vi "AssertDisable.vi"() -> (15 "error out":errorcluster)   [LabVIEW 2016, in "DronaTest.lvlib"]
uses:
  DronaTest.lvlib
  APIs/Stimulus/ControlValue/ValueSignalByPathString.vi
  APIs/Assert/AssertControlDisable/AssertDisabled.vi
  APIs/Assert/AssertControlDisable/AssertDisabledAndGrayedOut.vi
  APIs/Assert/AssertControlDisable/AssertEnabled.vi
  <vilib>/addons/_JKI Toolkits/Caraya/classes/Test/Test.lvclass
  Drona.lvlib
  APIs/Stimulus/ControlValue/ControlValue.lvlib
  APIs/Assert/AssertControlDisable/AssertControlDisable.lvlib
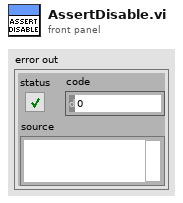
[diagram p1: front panel]
types:
  T1 = enum8{"Enabled", "Disabled", "Disabled and Grayed Out"}
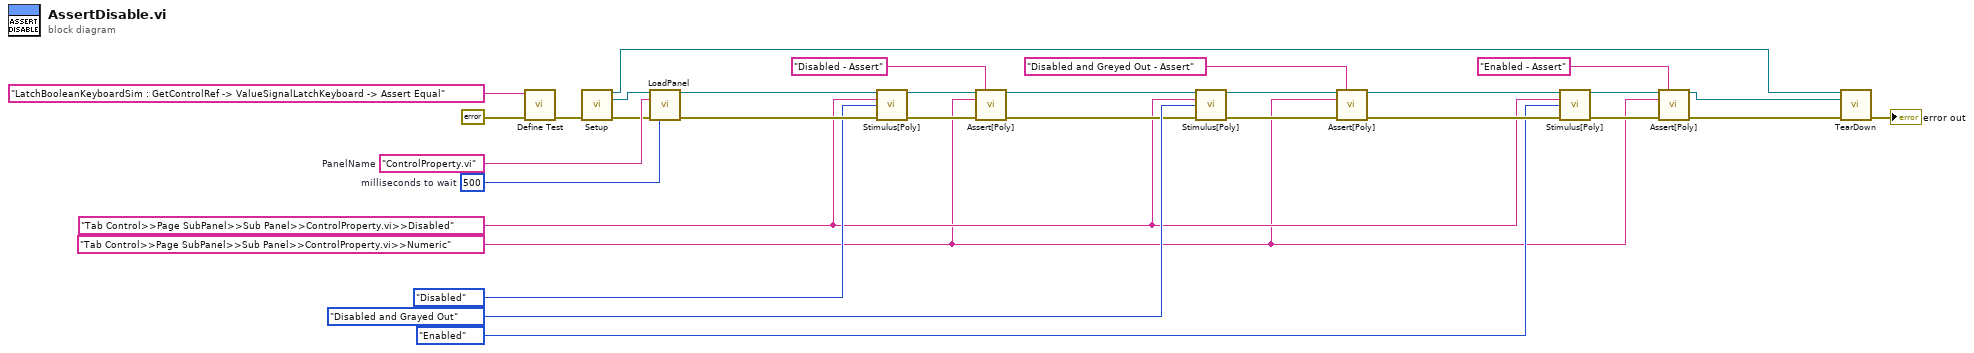
[diagram p0: block diagram]
diagram:
  w24 = u32 500  # milliseconds to wait
  w9 = "Tab Control>>Page SubPanel>>Sub Panel>>ControlProperty.vi>>Numeric" ("Control Path")
  w10 = "Tab Control>>Page SubPanel>>Sub Panel>>ControlProperty.vi>>Disabled" ("Control Path")
  w30 = "ControlProperty.vi"  # PanelName
  n1 = call <vilib>:"Define Test.vi"("error in (no error)"=errorcluster {"status"=FALSE, "code"=0, "source"=""}, "Label (VI Title)"="LatchBooleanKeyboardSim : GetControlRef -> ValueSignalLatchKeyboard -> Assert Equal") -> ("error out"=w5:errorcluster)  [unwired: 9 in]
  n2 = call "Setup.vi"("error in (no error)"=w5) -> ("Application Ref"=w1:refnum<vi>, "VI out"=w6:refnum<vi>, "error out"=w7:errorcluster)  [unwired: 12 in]
  n3 = call "LoadPanel.vi"("VI in"=w6, "Panel Name"=w30, "error in (no error)"=w7, "milliseconds to wait"=w24) -> ("VI out"=w28:refnum<vi>, "error out"=w25:errorcluster)  [unwired: 10 in]
  n4 = call-poly "Stimulus[Poly].vi"("VI Reference In"=w28, "Control Path"=w10, "Value (Signaling)"=T1."Disabled" ("Disabled"), "error in"=w25) -> ("VI Reference Out"=w27:refnum<vi>, "error out"=w29:errorcluster)  [unwired: 10 in]
  n5 = call-poly "Assert[Poly].vi"("VI Reference In"=w27, "Test Label"="Disabled - Assert" ("string"), "Control Path"=w9, "Error In"=w29) -> ("VI Reference Out"=w18:refnum<vi>, "Error Out"=w17:errorcluster)  [unwired: 10 in]
  n6 = call-poly "Stimulus[Poly].vi"("VI Reference In"=w18, "Control Path"=w10, "Value (Signaling)"=T1."Disabled and Grayed Out" ("Disabled"), "error in"=w17) -> ("VI Reference Out"=w20:refnum<vi>, "error out"=w19:errorcluster)  [unwired: 10 in]
  n7 = call-poly "Assert[Poly].vi"("VI Reference In"=w20, "Test Label"="Disabled and Greyed Out - Assert" ("string"), "Control Path"=w9, "Error In"=w19) -> ("VI Reference Out"=w12:refnum<vi>, "Error Out"=w13:errorcluster)  [unwired: 10 in]
  n8 = call-poly "Stimulus[Poly].vi"("VI Reference In"=w12, "Control Path"=w10, "Value (Signaling)"=T1."Enabled" ("Disabled"), "error in"=w13) -> ("VI Reference Out"=w15:refnum<vi>, "error out"=w16:errorcluster)  [unwired: 10 in]
  n9 = call-poly "Assert[Poly].vi"("VI Reference In"=w15, "Test Label"="Enabled - Assert" ("string"), "Control Path"=w9, "Error In"=w16) -> ("VI Reference Out"=w2:refnum<vi>, "Error Out"=w3:errorcluster)  [unwired: 10 in]
  n10 = call "TearDown.vi"("Application Ref"=w1, "VI in"=w2, "error in (no error)"=w3) -> ("error out"=→"error out":errorcluster)  [unwired: 12 in]
